vi "GetActualSteerAngles.vi"(10 "Zero Relative Encoder":bool, 11 "Relative Encoders?":bool) -> (3 "Robot Motion Commands":T1)   [LabVIEW 2019]
doc: "Input: \nName: Relative Encoders? Type: Boolean Default: F (F=absolute, T=relative)\nName: Zero Relative Encoder Type: Boolean Default: F\n\nOutput: \nName: Actual Angles Type: Robot Pivot Motion Commands\n\nPurpose: \nTo get the actual angles from the encoders in units of degrees and align the neutral angle orientation with the frame on the robot\n\nAlgorithm: \nGet the steer angle encoder objects using the corresponding names found in the begin function. Different objects and functions will be needed if relative or absolute encoders are used. \n\nIf Relative Encoders input is False, get the absolute encoder objects and use the appropriate functions to read the encoder channels and convert to angle in degrees. Values should be between -180 and +180. Hard coded offsets should be used to align the motors with the frame and set that particular rotation as 0 degrees. Each encoder will require a different offset value. Bundle values into appropriate ‘Steer Angle (deg)’ in the Robot Pivot Motion Commands cluster.\n\nIf Relative Encoders input is True, get the relative encoder objects and use the appropriate functions to read the encoder channels and convert to angle in degrees. Values should be between -180 and +180. Bundle values into appropriate ‘Steer Angle (deg)’ in the Robot Pivot Motion Commands cluster.\n\nIf the Zero Relative Encoder input is True then get the relative encoder objects and use the appropriate functions to Reset all encoder channels."
uses:
  Controls/Robot Pivot Motion Commands.ctl
  Controls/Pivot Motor Commands.ctl
  Controls/Robot Drive Mode.ctl
  <vilib>/Rock Robotics/Network Tables/NT Write Numeric Array.vi
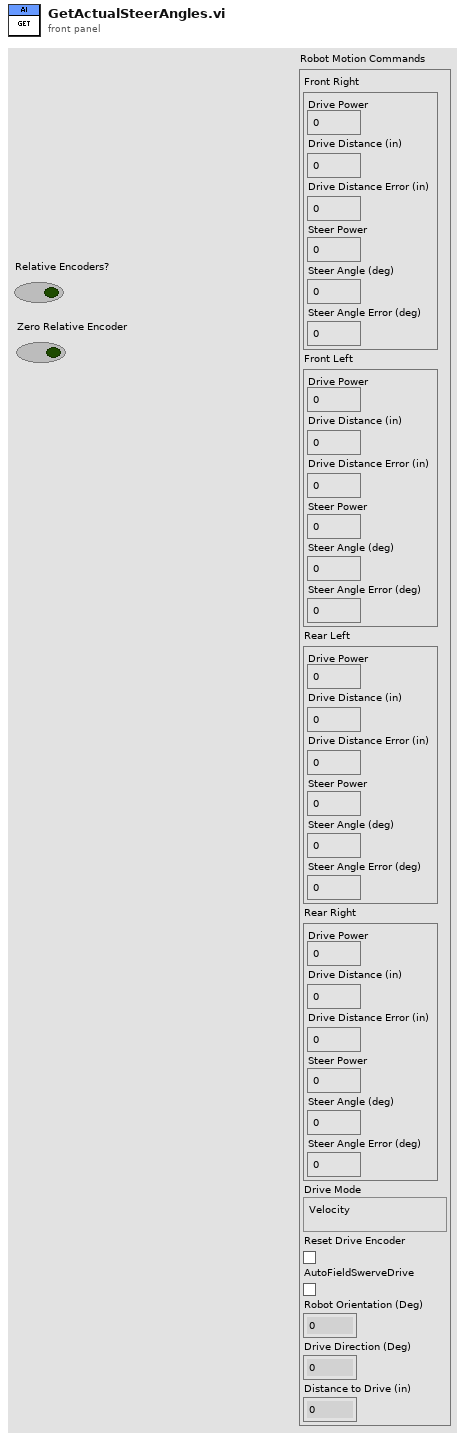
[diagram p1: front panel]
types:
  T1 = typedef "Robot Pivot Motion Commands.ctl" = cluster{"Front Right":T2, "Front Left":T2, "Rear Left":T2, "Rear Right":T2, "Drive Mode":T3, "Reset Drive Encoder":bool, "AutoFieldSwerveDrive":bool, "Robot Orientation (Deg)":dbl, "Drive Direction (Deg)":dbl, "Distance to Drive (in)":dbl}
  T2 = typedef "Pivot Motor Commands.ctl" = cluster{"Drive Power":dbl, "Drive Distance (in)":dbl, "Drive Distance Error (in)":dbl, "Steer Power":dbl, "Steer Angle (deg)":dbl, "Steer Angle Error (deg)":dbl}
  T3 = typedef "Robot Drive Mode.ctl" = enum16{"Velocity", "Distance"}
  T4 = typedef "WPI_AnalogChannelDevRef.ctl" = cluster{"DevStatus":errorcluster, "Analog Channel":T5}
  T5 = typedef "FPGA_AIChannel.ctl" = enum8{"AI 0", "AI 1", "AI 2", "AI 3", "AI MXP 0", "AI MXP 1", "AI MXP 2", "AI MXP 3", "Invalid"}
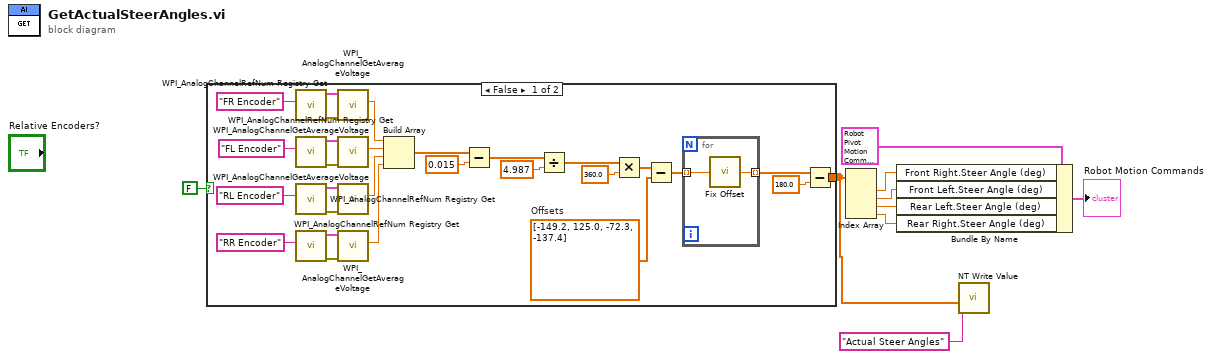
[diagram p0: block diagram]
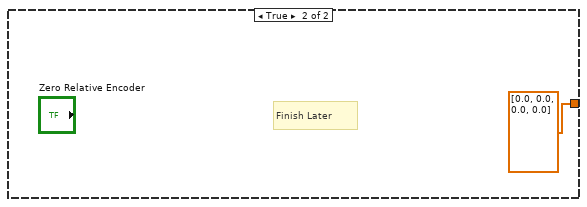
[diagram p2: hidden frame]
diagram:
  n1 = case shown="False" FALSE {
    tunnel: [w11 dbl[] [0.0, 0.0, 0.0, 0.0]] -> w2
    frame False {
      w14 = dbl[] [-149.2, 125.0, -72.3, -137.4]  # Offsets
      n2 = call <vilib>:"WPI_AnalogChannelRefNum Registry Get.vi"("refnum name"="FR Encoder") -> ("error out"=w37:errorcluster, "AIDeviceRef"=w36:T4)  [unwired: 9 in]
      n3 = call <vilib>:"WPI_AnalogChannelRefNum Registry Get.vi"("refnum name"="FL Encoder") -> ("error out"=w34:errorcluster, "AIDeviceRef"=w33:T4)  [unwired: 9 in]
      n4 = call <vilib>:"WPI_AnalogChannelRefNum Registry Get.vi"("refnum name"="RL Encoder") -> ("error out"=w31:errorcluster, "AIDeviceRef"=w30:T4)  [unwired: 9 in]
      n5 = call <vilib>:"WPI_AnalogChannelRefNum Registry Get.vi"("refnum name"="RR Encoder") -> ("error out"=w28:errorcluster, "AIDeviceRef"=w27:T4)  [unwired: 9 in]
      n6 = call <vilib>:"WPI_AnalogChannelGetAverageVoltage.vi"("error in (no error)"=w37, "AIDeviceRef"=w36) -> ("Voltage"=w18:dbl)  [unwired: 7 in, 2 out]
      n7 = call <vilib>:"WPI_AnalogChannelGetAverageVoltage.vi"("error in (no error)"=w34, "AIDeviceRef"=w33) -> ("Voltage"=w17:dbl)  [unwired: 7 in, 2 out]
      n8 = call <vilib>:"WPI_AnalogChannelGetAverageVoltage.vi"("error in (no error)"=w31, "AIDeviceRef"=w30) -> ("Voltage"=w16:dbl)  [unwired: 7 in, 2 out]
      n9 = call <vilib>:"WPI_AnalogChannelGetAverageVoltage.vi"("error in (no error)"=w28, "AIDeviceRef"=w27) -> ("Voltage"=w15:dbl)  [unwired: 7 in, 2 out]
      n10 = Build Array(w18, w17, w16, w15) -> (w10:dbl[])
      n11 = Subtract(x=w10, y=0.015) -> (x-y=w24:dbl[])
      n12 = Divide(x=w24, y=4.987) -> (x/y=w22:dbl[])
      n13 = Multiply(x=w22, y=360.0) -> (x*y=w20:dbl[])
      n14 = Subtract(x=w20, y=w14) -> (x-y=w13:dbl[])
      n15 = for {
        tunnel: w13 -> [w39] mode=indexing
        tunnel: [w38] -> w12 mode=indexing
        n16 = call "Fix Offset.vi"("Input Angle"=w39) -> ("Output Angle"=w38:dbl)
      }
      n17 = Subtract(x=w12, y=180.0) -> (x-y=w11:dbl[])
    }
    frame True {
      # "Finish Later"
    }
  }
  n18 = Index Array(array=w2) -> (element #1=w7:dbl, element #2=w6:dbl, element #3=w5:dbl, element #4=w4:dbl)  [unwired: 4 in]
  n19 = Bundle By Name(cluster=T1 {"Front Right"={"Drive Power"=0.0, "Drive Distance (in)"=0.0, "Drive Distance Error (in)"=0.0, "Steer Power"=0.0, "Steer Angle (deg)"=0.0, "Steer Angle Error (deg)"=0.0}, "Front Left"={"Drive Power"=0.0, "Drive Distance (in)"=0.0, "Drive Distance Error (in)"=0.0, "Steer Power"=0.0, "Steer Angle (deg)"=0.0, "Steer Angle Error (deg)"=0.0}, "Rear Left"={"Drive Power"=0.0, "Drive Distance (in)"=0.0, "Drive Distance Error (in)"=0.0, "Steer Power"=0.0, "Steer Angle (deg)"=0.0, "Steer Angle Error (deg)"=0.0}, "Rear Right"={"Drive Power"=0.0, "Drive Distance (in)"=0.0, "Drive Distance Error (in)"=0.0, "Steer Power"=0.0, "Steer Angle (deg)"=0.0, "Steer Angle Error (deg)"=0.0}, "Drive Mode"=enum."Velocity", "Reset Drive Encoder"=FALSE, "AutoFieldSwerveDrive"=FALSE, "Robot Orientation (Deg)"=0.0, "Drive Direction (Deg)"=0.0, "Distance to Drive (in)"=0.0} ("Robot Motion Commands"), "Front Right.Steer Angle (deg)"=w7, "Front Left.Steer Angle (deg)"=w6, "Rear Left.Steer Angle (deg)"=w5, "Rear Right.Steer Angle (deg)"=w4) -> (→"Robot Motion Commands":T1)
  n20 = call-poly <vilib>:"NT Write Value.vi"("Numeric Array"=w2, "Name"="Actual Steer Angles") -> ()  [unwired: 9 in, 1 out]
